vi "Wave-Write Chunk.vi"(8 "error in (no error)":errorcluster, 10 "ID":string, 11 "refnum":refnum<file>) -> (0 "error out":errorcluster, 1 "EOF?":bool, 2 "chunk info":T1, 3 "refnum out":refnum<file>)   [LabVIEW 2015]
uses:
  Wave-Chunk Info.ctl
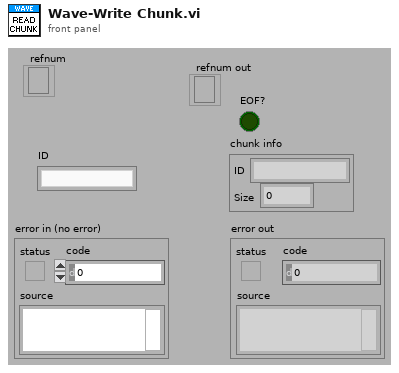
[diagram p1: front panel]
types:
  T1 = typedef "Wave-Chunk Info.ctl" = cluster{"ID":string, "Size":u32}
  T2 = enum16{"big-endian, network order", "native, host order", "little-endian"}
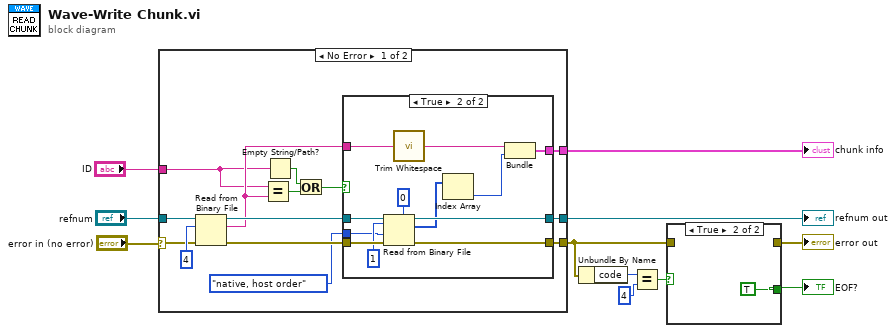
[diagram p0: block diagram]
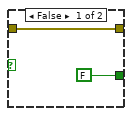
[diagram p2: hidden frame]
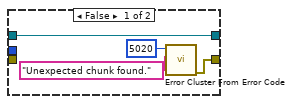
[diagram p3: hidden frame]
diagram:
  n1 = case shown="No Error" "error in (no error)" {
    selector: "error in (no error)" -> [w17 w42]
    tunnel: "refnum" -> [w25 w43]
    tunnel: [w21 _] -> w10
    tunnel: [w20 w43] -> w9
    tunnel: [w19 w42] -> w1
    tunnel: "ID" -> [w13 _]
    frame No Error {
      n2 = Read from Binary File(8:w17, 10:4, 11:w25) -> (0:w23:errorcluster, 2:w14:string, 3:w22:refnum<file>)  [unwired: 3 in, 1 out]
      n3 = Equal?(x=w13, y=w14) -> (x = y?=w18:bool)
      n4 = Empty String/Path?(string/path=w13) -> (empty?=w15:bool)
      n5 = Or(x=w15, y=w18) -> (x .or. y?=w16:bool)
      n6 = case shown="True" w16 {
        tunnel: w23 -> [_ w41]
        tunnel: w22 -> [w29 w40]
        tunnel: [_ w30] -> w21
        tunnel: [w29 w38] -> w20
        tunnel: [w28 w37] -> w19
        tunnel: w14 -> [_ w36]
        tunnel: T2."native, host order" ("byte order (0:big-endian, network order)") -> [_ w34]
        frame False {
          n7 = call <vilib>:"Error Cluster From Error Code.vi"("error message (\"\")"="Unexpected chunk found." ("source"), "error code (0)"=5020) -> ("error out"=w28:errorcluster)  [unwired: 7 in]
        }
        frame True {
          n8 = Read from Binary File(5:u32 0, 8:w41, 9:w34, 10:1, 11:w40) -> (0:w37:errorcluster, 2:w32:u32[], 3:w38:refnum<file>)  [unwired: 1 in, 1 out]
          n9 = call <vilib>:"Trim Whitespace.vi"("string"=w36) -> ("trimmed string"=w35:string)  [unwired: 1 in]
          n10 = Index Array(array=w32) -> (element=w31:u32)  [unwired: 1 in]
          n11 = Bundle("trimmed string"=w35, w31) -> (w30:cluster{"trimmed string":string, u32})  [unwired: 1 in]
        }
      }
    }
    frame Error {
    }
  }
  "refnum out" <- w9
  "chunk info" <- w10
  n12 = Unbundle By Name(w1) -> ("code"=w4:i32)
  n13 = Equal?(x=w4, y=4) -> (x = y?=w2:bool)
  n14 = case shown="True" w2 {
    tunnel: [w44 _] -> w6
    tunnel: [FALSE TRUE] -> w5
    tunnel: w1 -> [w44 _]
    frame False {
    }
    frame True {
    }
  }
  "error out" <- w6
  "EOF?" <- w5
